vi "UpdateLaserParameters.vi"(7 "error in":errorcluster) -> (18 "interlock":bool, 20 "em":bool, 26 "ToShell":string, 27 "error out":errorcluster)   [LabVIEW 2011]
uses:
  Variables/LaserParameter.vi
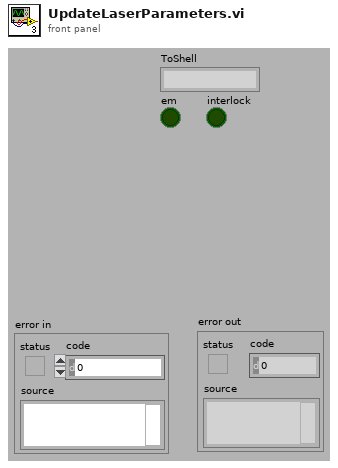
[diagram p1: front panel]
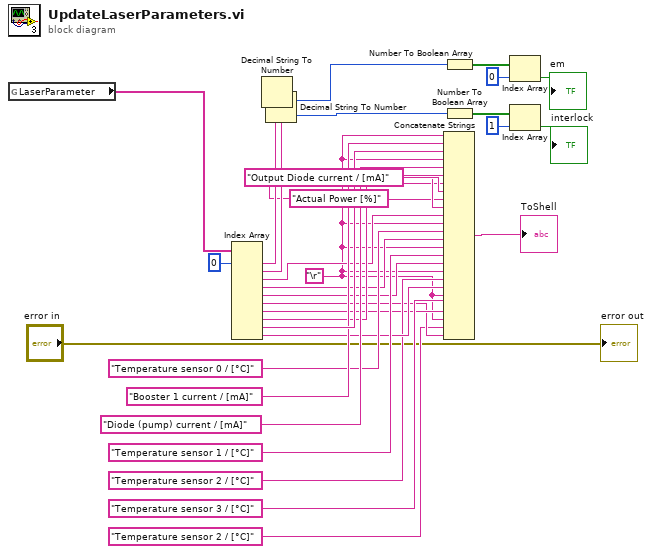
[diagram p0: block diagram]
diagram:
  w8 = "\r"
  n1 = global read "LaserParameter.vi" "LaserParameter"() -> (w4:string[])
  n2 = Index Array(array=w4, index #1=0 ("index")) -> (element #1=w32:string, element #2=w31:string, element #3=w17:string, element #4=w15:string, element #5=w13:string, element #6=w7:string, element #7=w9:string, element #8=w20:string, element #9=w23:string, element #10=w12:string)  [unwired: 9 in]
  n3 = Decimal String To Number(string=w32) -> (number=w30:i32)  [unwired: 2 in, 1 out]
  n4 = Decimal String To Number(string=w31) -> (number=w5:i32)  [unwired: 2 in, 1 out]
  n5 = Concatenate Strings(w8, "Booster 1 current / [mA]" ("string"), w23, w8, "Diode (pump) current / [mA]" ("string"), w20, w8, "Output Diode current / [mA]" ("string"), w8, "Actual Power [%]" ("string"), w17, w8, "Temperature sensor 0 / [°C]" ("string"), w15, w8, "Temperature sensor 1 / [°C]" ("string"), w13, w8, "Temperature sensor 2 / [°C]" ("string"), w12, w8, "Temperature sensor 3 / [°C]" ("string"), w9, w8, "Temperature sensor 2 / [°C]" ("string"), w7) -> (→"ToShell":string)
  n6 = Number To Boolean Array(number=w30) -> (Boolean array=w29:bool[])
  n7 = Number To Boolean Array(number=w5) -> (Boolean array=w26:bool[])
  n8 = Index Array(array=w29, index=0) -> (element=→"em":bool)
  n9 = Index Array(array=w26, index=1) -> (element=→"interlock":bool)
  "error out" <- "error in"
